vi "Main Abstraction Level 1.vi"() -> ()   [LabVIEW 2023]
doc: "This is one of the levels of abstract design along the timeline leading to the goal of a complete measurement application."
uses:
  messages/MeasureAndLogMessage.lvclass/MeasureAndLogMessage.ctl
  <extravilib>/ChannelInstances/Lossy Stream-a[.](wfm(dbl))/Read With Abort.vi
  <extravilib>/ChannelInstances/Stream-str/Read With Abort.vi
  <extravilib>/ChannelInstances/Messenger-class'MeasureAndLogMessage'/Write With Abort.vi
  <extravilib>/ChannelInstances/Lossy Stream-a[.](wfm(dbl))/EndpointRead.vi
  <extravilib>/ChannelInstances/Stream-str/EndpointRead.vi
  <extravilib>/ChannelInstances/Stream-a[.](wfm(dbl))/Instantiate.vi
  <extravilib>/ChannelInstances/Tag-path/Instantiate.vi
  <extravilib>/ChannelInstances/Stream-str/Instantiate.vi
  <extravilib>/ChannelInstances/Stream-str/)Channel.vi
  <resource>/ChannelSupport/_ChannelSupport/WaitIfNeeded.vi
  <extravilib>/ChannelInstances/Lossy Stream-a[.](wfm(dbl))/Instantiate.vi
  <extravilib>/ChannelInstances/Lossy Stream-a[.](wfm(dbl))/)Channel.vi
  <extravilib>/ChannelInstances/Messenger-class'MeasureAndLogMessage'/Instantiate.vi
  <extravilib>/ChannelInstances/Messenger-class'MeasureAndLogMessage'/Endpoint.vi
  messages/MeasureAndLogMessage.lvclass
  <extravilib>/ChannelInstances/Stream-str.lvlib
  <extravilib>/ChannelInstances/Lossy Stream-a[.](wfm(dbl)).lvlib
  <extravilib>/ChannelInstances/Messenger-class'MeasureAndLogMessage'.lvlib
panel:
  in  "Exit flag":bool
  in  "Record":bool
  in  "Stop":bool
  out "Data":waveform(dbl)[](graph)
  out "Status":string
  in  "Settings":bool
  in  "Start":bool
  in  "Exit":bool
  # "Continuous Measurement Data Logger"
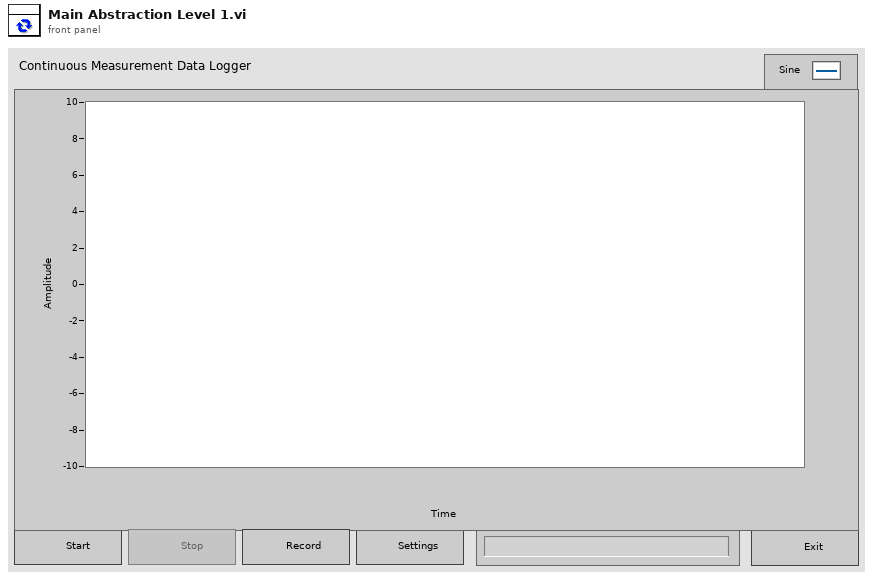
[diagram p1: front panel]
types:
  T1 = typedef "Measure and Log Settings.ctl" = cluster{"sample rate":dbl, "input range":dbl, "logfile path":path, "Simulated Signal":cluster{"signal type":T2, "frequency":dbl, "amplitude":dbl}}
  T2 = typedef "Simulated Signal Type.ctl" = enum16{"Sine Wave", "Square Wave with Noise"}
  T3 = enum8{"Enabled", "Disabled", "Disabled and Grayed Out"}
  T4 = typedef "Messenger-class'MeasureAndLogMessage'.lvlib/))Channel.ctl" = refnum<queue>
  T5 = typedef "Stream-a[.](wfm(dbl)).lvlib/)Channel.ctl" = refnum<queue>
  T6 = typedef "Tag-path.lvlib/))Channel.ctl" = refnum<queue>
  T7 = typedef "Stream-str.lvlib/)Channel.ctl" = refnum<queue>
  T8 = typedef "Lossy Stream-a[.](wfm(dbl)).lvlib/)Channel.ctl" = refnum<queue>
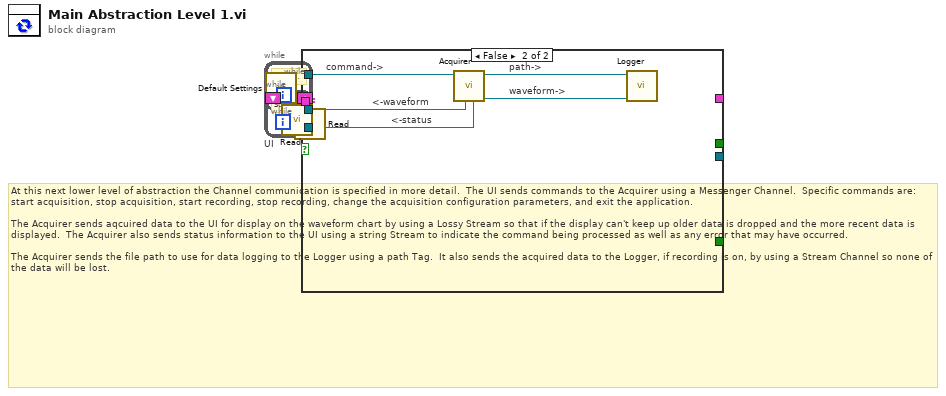
[diagram p0: block diagram]
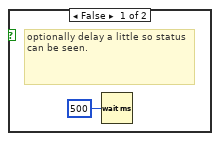
[diagram p2: hidden frame]
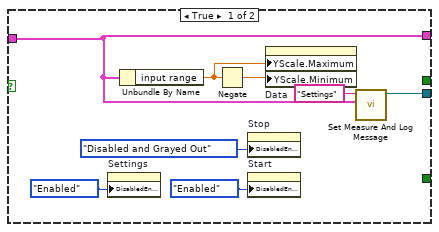
[diagram p3: hidden frame]
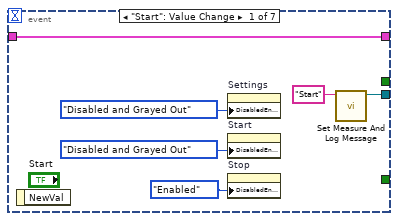
[diagram p4: hidden frame]
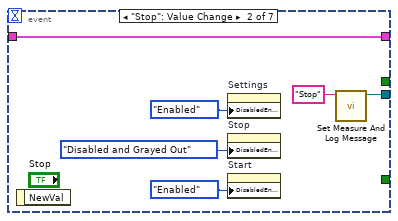
[diagram p5: hidden frame]
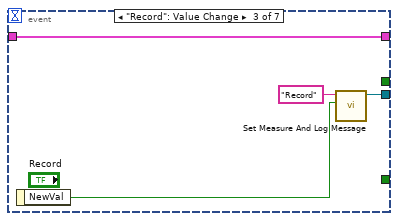
[diagram p6: hidden frame]
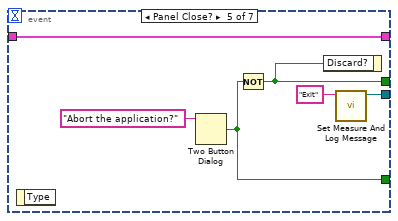
[diagram p7: hidden frame]
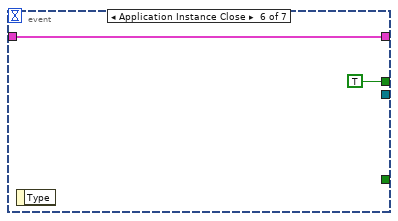
[diagram p8: hidden frame]
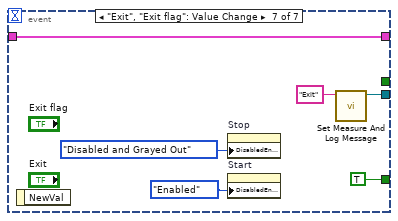
[diagram p9: hidden frame]
diagram:
  # "At this next lower level of abstraction the Channel communication is specified in more detail.  The UI sends commands to the Acquirer using a Messenger Channel.  Specific commands are: start acquisition, stop acquisition, start recording, stop recording, change the acquisition configuration parameters, and exit the application.\n\nThe Acquirer sends aqcuired data to the UI for display on the waveform chart by using a Lossy Stream so that if the display can't keep up older data is dropped and the more recent data is displayed.  The Acquirer also sends status information to the UI using a string Stream to indicate the command being processed as well as any error that may have occurred.\n\nThe Acquirer sends the file path to use for data logging to the Logger using a path Tag.  It also sends the acquired data to the Logger, if recording is on, by using a Stream Channel so none of the data will be lost."
  # "waveform->"
  # "path->"
  # "<-status"
  # "<-waveform"
  # "command->"
  n1 = while "UI" {
    i -> [w8]
    stop <- w7 stop-if-true
    n2 = Greater Than 0?(x=w8) -> (x > 0?=w7:bool)
  }
  n3 = call "Default Settings.vi"() -> ("default settings"=w5:T1)
  n4 = while "Event Handling Loop" {
    tunnel: [w11] -> w6
    shift-right: [w14] -> _
    shift-left: w5 -> [w13]
    stop <- w15 stop-if-true
    # "Event Handling Loop"
    n5 = First Call?() -> (First Call?: T/F=w12:bool)
    n6 = case shown="False" w12 {
      tunnel: [_ w28] -> w15
      tunnel: [w22 w27] -> w14
      tunnel: w13 -> [w22 w26]
      tunnel: [w18 w25] -> w10
      tunnel: [_ w24] -> w9
      frame True {
        n7 = property on="Settings" class="Bool"("DisabledEnum"=T3."Enabled" ("Disabled")) -> ()  [unwired: 2 in, 2 out]
        n8 = Unbundle By Name(w22) -> ("input range"=w16:dbl)
        n9 = Negate(x=w16) -> (-x=w17:dbl)
        n10 = property on="Stop" class="Bool"("DisabledEnum"=T3."Disabled and Grayed Out" ("Disabled")) -> ()  [unwired: 2 in, 2 out]
        n11 = property on="Start" class="Bool"("DisabledEnum"=T3."Enabled" ("Disabled")) -> ()  [unwired: 2 in, 2 out]
        n12 = property on="Data" class="WFChart (strict)"("YScale.Maximum"=w16, "YScale.Minimum"=w17) -> ()  [unwired: 2 in, 2 out]
        n13 = call "Set Measure And Log Message.vi"("args"=w22, "command"="Settings") -> ("MyMessage"=w18:refnum<class "MeasureAndLogMessage.lvclass">)  [unwired: 9 in]
      }
      frame False {
        n14 = event shown="[3] \"Settings\": Value Change" {
          selector: _ -> [_ _ _ _ _ _ _]
          dyn-events: _ -> [_ _ _ _ _ _ _]
          timeout: _ -> [_ _ _ _ _ _ _]
          tunnel: [_ _ _ _ w53 _ TRUE] -> w28
          tunnel: [w30 w36 w42 w50 w56 w59 w61] -> w27
          tunnel: w26 -> [w30 w36 w42 w51 w56 w59 w61]
          tunnel: [w29 w35 w41 w49 w54 _ w60] -> w25
          tunnel: [_ _ _ w47 w52 TRUE ("cancelled") _] -> w24
          event "Start": Value Change {
            n15 = event-data() -> ()  [unwired: 1 in, 1 out]
            n16 = property on="Settings" class="Bool"("DisabledEnum"=T3."Disabled and Grayed Out" ("Disabled")) -> ()  [unwired: 2 in, 2 out]
            n17 = property on="Start" class="Bool"("DisabledEnum"=T3."Disabled and Grayed Out" ("Disabled")) -> ()  [unwired: 2 in, 2 out]
            n18 = property on="Stop" class="Bool"("DisabledEnum"=T3."Enabled" ("Disabled")) -> ()  [unwired: 2 in, 2 out]
            n19 = call "Set Measure And Log Message.vi"("command"="Start") -> ("MyMessage"=w29:refnum<class "MeasureAndLogMessage.lvclass">)  [unwired: 10 in]
          }
          event "Stop": Value Change {
            n20 = event-data() -> ()  [unwired: 1 in, 1 out]
            n21 = property on="Settings" class="Bool"("DisabledEnum"=T3."Enabled" ("Disabled")) -> ()  [unwired: 2 in, 2 out]
            n22 = property on="Stop" class="Bool"("DisabledEnum"=T3."Disabled and Grayed Out" ("Disabled")) -> ()  [unwired: 2 in, 2 out]
            n23 = property on="Start" class="Bool"("DisabledEnum"=T3."Enabled" ("Disabled")) -> ()  [unwired: 2 in, 2 out]
            n24 = call "Set Measure And Log Message.vi"("command"="Stop") -> ("MyMessage"=w35:refnum<class "MeasureAndLogMessage.lvclass">)  [unwired: 10 in]
          }
          event "Record": Value Change {
            n25 = event-data() -> ("NewVal"=w43:bool)  [unwired: 1 in]
            n26 = call "Set Measure And Log Message.vi"("args"=w43, "command"="Record") -> ("MyMessage"=w41:refnum<class "MeasureAndLogMessage.lvclass">)  [unwired: 9 in]
          }
          event "Settings": Value Change {
            n27 = event-data() -> ()  [unwired: 1 in, 1 out]
            n28 = call "Settings Dialog.vi"("settings in"=w51) -> ("cancelled"=w47:bool, "settings out"=w50:T1)  [unwired: 9 in]
            n29 = Unbundle By Name(w50) -> ("input range"=w45:dbl)
            n30 = Negate(x=w45) -> (-x=w46:dbl)
            n31 = property on="Data" class="WFChart (strict)"("YScale.Maximum"=w45, "YScale.Minimum"=w46) -> ()  [unwired: 2 in, 2 out]
            n32 = call "Set Measure And Log Message.vi"("args"=w50, "command"="Settings") -> ("MyMessage"=w49:refnum<class "MeasureAndLogMessage.lvclass">)  [unwired: 9 in]
          }
          event Panel Close? {
            n33 = event-data() -> ()  [unwired: 1 in, 1 out]
            n34 = Two Button Dialog(message="Abort the application?") -> (T button?=w53:bool)  [unwired: 2 in]
            n35 = Not(x=w53) -> (.not. x?=w52:bool)
            n36 = event-data("Discard?"=w52) -> ()  [unwired: 1 in, 1 out]
            n37 = call "Set Measure And Log Message.vi"("command"="Exit") -> ("MyMessage"=w54:refnum<class "MeasureAndLogMessage.lvclass">)  [unwired: 10 in]
          }
          event Application Instance Close {
            n38 = event-data() -> ()  [unwired: 1 in, 1 out]
          }
          event "Exit", "Exit flag": Value Change {
            n39 = event-data() -> ()  [unwired: 1 in, 1 out]
            n40 = property on="Stop" class="Bool"("DisabledEnum"=T3."Disabled and Grayed Out" ("Disabled")) -> ()  [unwired: 2 in, 2 out]
            n41 = property on="Start" class="Bool"("DisabledEnum"=T3."Enabled" ("Disabled")) -> ()  [unwired: 2 in, 2 out]
            n42 = call "Set Measure And Log Message.vi"("command"="Exit") -> ("MyMessage"=w60:refnum<class "MeasureAndLogMessage.lvclass">)  [unwired: 10 in]
          }
        }
      }
    }
    n43 = case shown="False" w9 {
      tunnel: [w67 _] -> w11
      tunnel: w10 -> [w66 _]
      frame False {
        n44 = call <extravilib>:"Write.vi"("element"=w66) -> ("channel"=w67:T4)  [unwired: 8 in, 2 out]
      }
      frame True {
      }
    }
  }
  n45 = call "Acquirer.vi"("command stream"=w6) -> ("wfm data stream"=w1:T5, "file path tag"=w2:T6, "status stream"=w3:T7, "wfm data lossy stream"=w4:T8)  [unwired: 7 in]
  n46 = while "Wfm Display Loop" {
    tunnel: w4 -> [w68]
    stop <- w70 stop-if-true
    # "Data Display Loop"
    n47 = call <extravilib>:"Read.vi"("channel"=w68) -> ("last element?"=w70:bool, "element"=→"Data":waveform(dbl)[])  [unwired: 5 in, 4 out]
  }
  n48 = while "Status Display Loop" {
    tunnel: w3 -> [w73]
    stop <- w71 stop-if-true
    # "Status Display Loop"
    n49 = call <extravilib>:"Read.vi"("channel"=w73) -> ("last element?"=w71:bool, "element"=→"Status":string)  [unwired: 6 in, 3 out]
    n50 = case shown="True" w71 {
      frame False {
        # "optionally delay a little so status can be seen."
        n51 = Wait (ms)(milliseconds to wait=u32 500) -> ()  [unwired: 1 out]
      }
      frame True {
        # "If the acquisition loop detects a fatal error and aborts be sure the event handling loop wakes up"
        n52 = property on="Exit flag" class="Bool (strict)"("Val(Sgnl)"=TRUE) -> ()  [unwired: 2 in, 2 out]
      }
    }
  }
  n53 = call "Logger.vi"("wfm data stream"=w1, "file path tag"=w2) -> ()  [unwired: 9 in, 1 out]
